vi "Measure Output.vi"(8 "error in (no error)":errorcluster, 11 "36234A in":refnum<class "36234A.lvclass">) -> (0 "error out":errorcluster, 1 "Current":dbl[](array[numeric]), 2 "Voltage":dbl[](array[numeric]), 3 "36234A out":refnum<class "36234A.lvclass">)   [LabVIEW 2019, in "36234A.lvlib" / "36234A.lvclass"]
doc: "Child classes must override this VI:\n\nThis VI is the device specific query of current and voltage measurements. \nThe return values are: \nVoltage Array - One voltage measurement per channel single channel supplies should only return a single array element\nCurrent Array - - One current measurement per channel single channel supplies should only return a single array element"
uses:
  Library/36234A.lvclass
  C:/Users/Public/Documents/Development/builds/Instruments/PowerSupply.lvlibp/Library/PowerSupply.lvclass
  builds/Instruments/PowerSupply.lvlibp/Private/Accessors/Read Number of Channels.vi
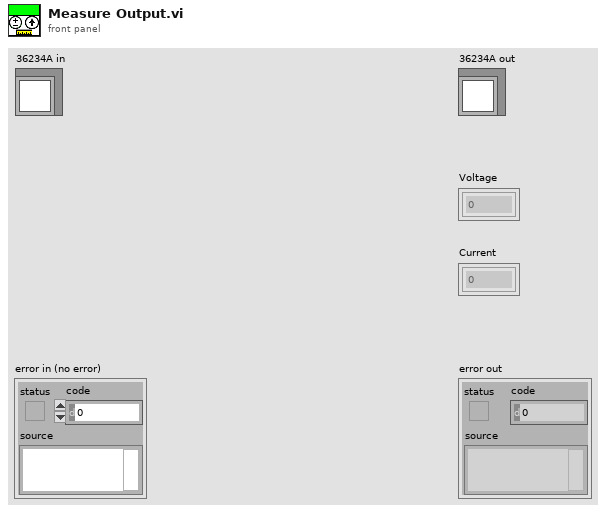
[diagram p1: front panel]
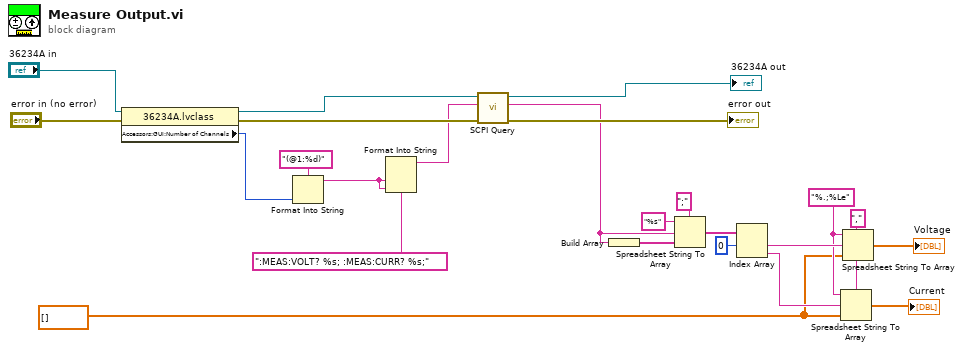
[diagram p0: block diagram]
diagram:
  w6 = dbl[] []
  w10 = "," ("delimiter (Tab)")
  w11 = "%.;%Le"
  n1 = property class="36234A.lvclass"(reference="36234A in", error in="error in (no error)") -> (reference out=w19:refnum<class "36234A.lvclass">, error out=w21:errorcluster, "Accessors:GUI:Number of Channels"=w1:i32)
  n2 = Format Into String(format string="(@1:%d)", w1) -> (resulting string=w2:string)  [unwired: 2 in, 1 out]
  n3 = Format Into String(format string=":MEAS:VOLT? %s; :MEAS:CURR? %s;", w2, w2) -> (resulting string=w16:string)  [unwired: 2 in, 1 out]
  n4 = call "SCPI Query.vi"("error in (no error)"=w21, "SCPI QUERY"=w16, "36234A in"=w19) -> ("error out"=→"error out":errorcluster, "read buffer"=w3:string, "36234A out"=→"36234A out":refnum<class "36234A.lvclass">)  [unwired: 6 in]
  n5 = Build Array(w3) -> (w7:string[])
  n6 = Spreadsheet String To Array(delimiter (Tab)=";", format string="%s", spreadsheet string=w3, array type (2D Dbl)=w7) -> (array=w12:string[])
  n7 = Index Array(array=w12, index #1=0 ("index")) -> (element #1=w14:string, element #2=w15:string)  [unwired: 1 in]
  n8 = Spreadsheet String To Array(delimiter (Tab)=w10, format string=w11, spreadsheet string=w15, array type (2D Dbl)=w6) -> (array=→"Current":dbl[])
  n9 = Spreadsheet String To Array(delimiter (Tab)=w10, format string=w11, spreadsheet string=w14, array type (2D Dbl)=w6) -> (array=→"Voltage":dbl[])
